vi "Update Frequency Scale.vi"(8 "Error In":errorcluster, 9 "Power Spectrum / PSD":cluster{"f0":dbl, "df":dbl, "magnitude":dbl[]}[](array[cluster]), 11 "Spectrogram Ref":refnum<vi>) -> (0 "Error Out":errorcluster, 2 "Frequency Scale Changed":bool)   [LabVIEW 2019]
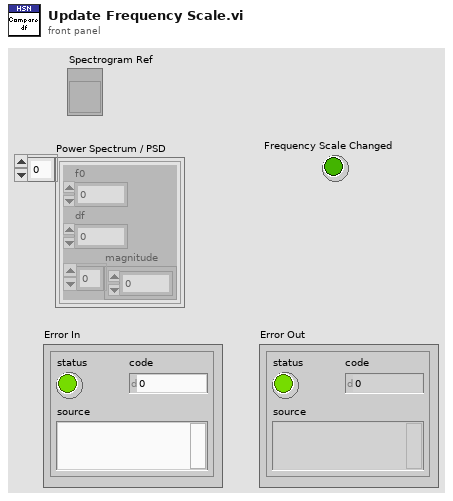
[diagram p1: front panel]
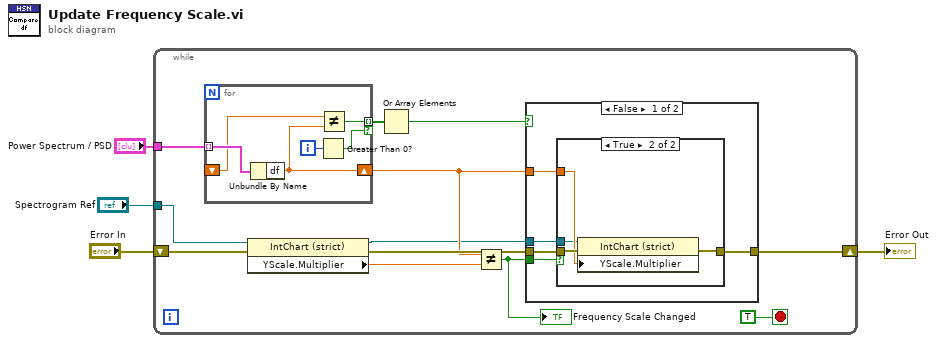
[diagram p0: block diagram]
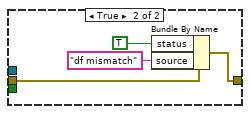
[diagram p3: hidden frame]
diagram:
  n1 = while {
    tunnel: "Power Spectrum / PSD" -> [w16]
    shift-right: [w13] -> w2
    shift-left: "Error In" -> [w11]
    tunnel: "Spectrogram Ref" -> [w6]
    stop <- TRUE stop-if-true
    n2 = for {
      tunnel: w16 -> [w36] mode=indexing
      tunnel: [w35] -> w14 mode=indexing if=w33
      shift-right: [w32] -> w7
      shift-left: _ -> [w31]
      i -> [w34]
      n3 = Unbundle By Name(w36) -> ("df"=w32:dbl)
      n4 = Greater Than 0?(x=w34) -> (x > 0?=w33:bool)
      n5 = Not Equal?(x=w31, y=w32) -> (x != y?=w35:bool)
    }
    n6 = property on="Property Node" class="IntChart (strict)"(reference=w6, error in=w11) -> (reference out=w5:refnum<vi>, error out=w9:errorcluster, "YScale.Multiplier"=w10:dbl)
    n7 = Or Array Elements(Boolean array=w14) -> (logical OR=w12:bool)
    n8 = Not Equal?(x=w7, y=w10) -> (x != y?=w8:bool)
    "Frequency Scale Changed" <- w8
    n9 = case shown="False" w12 {
      tunnel: [w21 w30] -> w13
      tunnel: w9 -> [w20 w28]
      tunnel: w8 -> [w19 _]
      tunnel: w7 -> [w18 _]
      tunnel: w5 -> [w17 _]
      frame False {
        n10 = case shown="True" w19 {
          tunnel: [w22 w26] -> w21
          tunnel: w20 -> [w22 w25]
          tunnel: w18 -> [_ w24]
          tunnel: w17 -> [_ w23]
          frame False {
          }
          frame True {
            n11 = property on="Property Node" class="IntChart (strict)"(reference=w23, error in=w25, "YScale.Multiplier"=w24) -> (error out=w26:errorcluster)  [unwired: 1 out]
          }
        }
      }
      frame True {
        n12 = Bundle By Name(cluster=w28, "status"=TRUE, "source"="df mismatch") -> (w30:errorcluster)
      }
    }
  }
  "Error Out" <- w2
